vi "setSettingsEventsManager.vi"(8 "error in (no error)":errorcluster, 10 "Tools.lvlib:Settings.lvlib:SettingsEventsManager.lvclass":refnum<class "SettingsEventsManager.lvclass">, 11 "CameraEventsManger.lvclass in":refnum<class "CameraEventsManger.lvclass">) -> (0 "error out":errorcluster, 3 "CameraEventsManger.lvclass out":refnum<class "CameraEventsManger.lvclass">)   [LabVIEW 2009, in "Tools.lvlib" / "Settings.lvlib" / "CameraEventsManger.lvclass"]
uses:
  CameraEventsManger.lvclass
  Tools/SettingsEventManager/SettingsEventsManager.lvclass
  CameraEventsManger.lvclass/CameraEventsManger.ctl
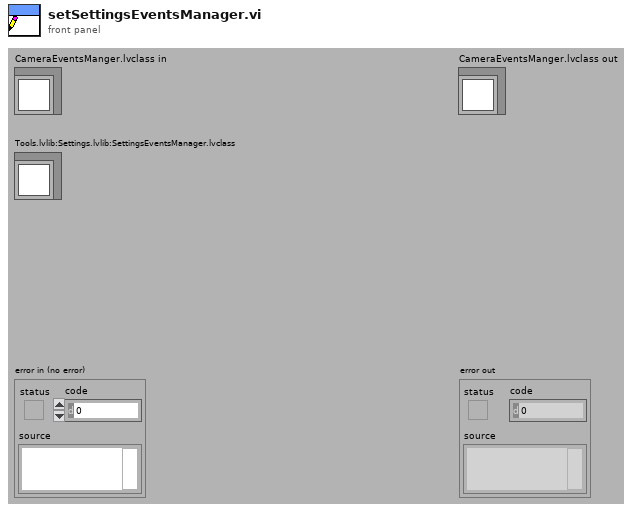
[diagram p1: front panel]
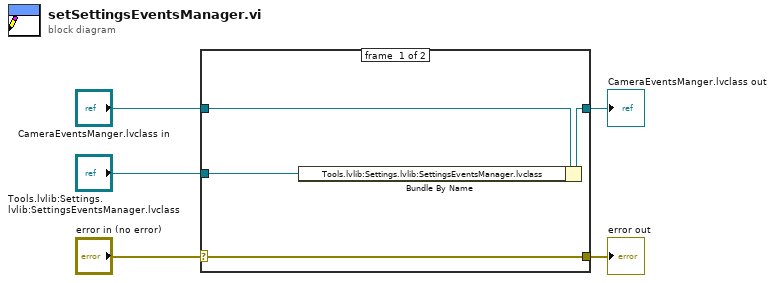
[diagram p0: block diagram]
diagram:
  n1 = case shown="No Error" "error in (no error)" {
    selector: "error in (no error)" -> [w9 w10]
    tunnel: [w9 w10] -> w4
    tunnel: [w7 w11] -> w2
    tunnel: "CameraEventsManger.lvclass in" -> [w8 w11]
    tunnel: "Tools.lvlib:Settings.lvlib:SettingsEventsManager.lvclass" -> [w6 _]
    frame #0 {
      n2 = Bundle By Name(cluster=w8, "Tools.lvlib:Settings.lvlib:SettingsEventsManager.lvclass"=w6) -> (w7:refnum<class "CameraEventsManger.lvclass">)
    }
    frame #1 {
    }
  }
  "error out" <- w4
  "CameraEventsManger.lvclass out" <- w2
